vi "Read_Element.vi"(8 "error in (no error)":errorcluster, 10 "Cell to Read":string="C2", 11 "Automation Refnum in":refnum<k7>) -> (0 "error out":errorcluster, 2 "Result":dbl, 3 "reference out":refnum<k7>)   [LabVIEW 2014]
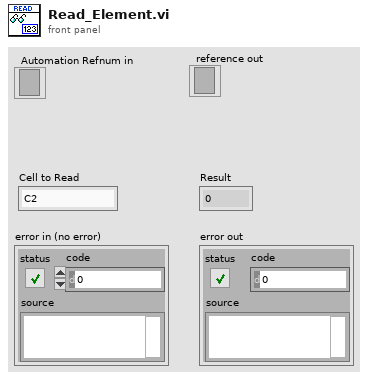
[diagram p1: front panel]
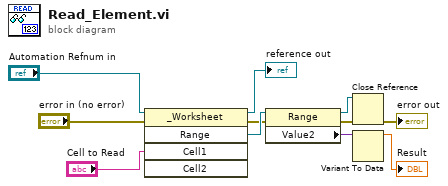
[diagram p0: block diagram]
diagram:
  n1 = invoke class="_Worksheet" method="Range"(reference="Automation Refnum in", error in="error in (no error)", "Cell1"="Cell to Read") -> (reference out=→"reference out":refnum<k7>, error out=w5:errorcluster, "Range"=w6:refnum<k7>)  [unwired: 2 in, 2 out]
  n2 = property class="Range"(reference=w6, error in=w5) -> (reference out=w3:refnum<k7>, error out=w2:errorcluster, "Value2"=w7:variant)
  n3 = Close Reference(reference=w3, error in (no error)=w2) -> (error out=→"error out":errorcluster)
  n4 = Variant To Data(Variant=w7) -> (data=→"Result":dbl)  [unwired: 2 in, 1 out]
